vi "DiffKinematics_toChassisSpeed.vi"(8 "TrackWidth_Meters":dbl, 10 "RightVelocity":dbl, 11 "LeftVelocity":dbl) -> (3 "CHASSIS Speed":T1)   [LabVIEW 2019, in "PathExecution_Library.lvlib"]
uses:
  PathExecution_Library.lvlib
  CHASSIS.ctl
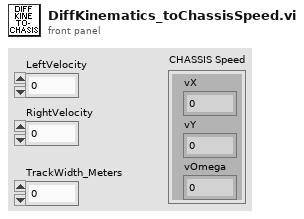
[diagram p1: front panel]
types:
  T1 = typedef "PathExecution_Library.lvlib/CHASSIS.ctl" = cluster{"vX":dbl, "vY":dbl, "vOmega":dbl}
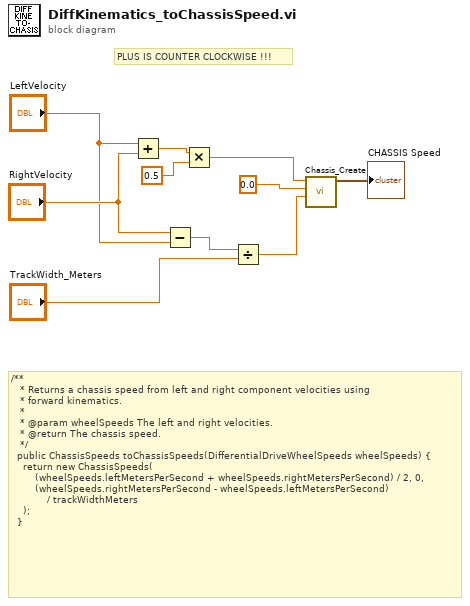
[diagram p0: block diagram]
diagram:
  # "PLUS IS COUNTER CLOCKWISE !!!"
  # "/**\n   * Returns a chassis speed from left and right component velocities using\n   * forward kinematics.\n   *\n   * @param wheelSpeeds The left and right velocities.\n   * @return The chassis speed.\n   */\n  public ChassisSpeeds toChassisSpeeds(DifferentialDriveWheelSpeeds wheelSpeeds) {\n    return new ChassisSpeeds(\n        (wheelSpeeds.leftMetersPerSecond + wheelSpeeds.rightMetersPerSecond) / 2, 0,\n        (wheelSpeeds.rightMetersPerSecond - wheelSpeeds.leftMetersPerSecond)\n            / trackWidthMeters\n    );\n  }"
  n1 = Add(x="LeftVelocity", y="RightVelocity") -> (x+y=w8:dbl)
  n2 = Subtract(x="RightVelocity", y="LeftVelocity") -> (x-y=w3:dbl)
  n3 = Multiply(x=w8, y=0.5) -> (x*y=w7:dbl)
  n4 = Divide(x=w3, y="TrackWidth_Meters") -> (x/y=w1:dbl)
  n5 = call "Chassis_Create.vi"("vAngular"=w1, "vY"=0.0, "vX"=w7) -> ("CHASSIS"=→"CHASSIS Speed":T1)  [unwired: 8 in]
